vi "简易计算器的制作(下).vi"() -> ()   [LabVIEW 2018]
panel:
  out "结果输出":dbl
  out "当前输入":string
  in  "?":bool
  in  "?":bool
  in  "?":bool
  in  "?":bool
  in  "?":bool
  in  "?":bool
  in  "?":bool
  in  "?":bool
  in  "?":bool
  in  "?":bool
  in  "?":bool
  in  "?":bool
  in  "?":bool
  in  "?":bool
  in  "?":bool
  in  "?":bool
  # "简易计算器"
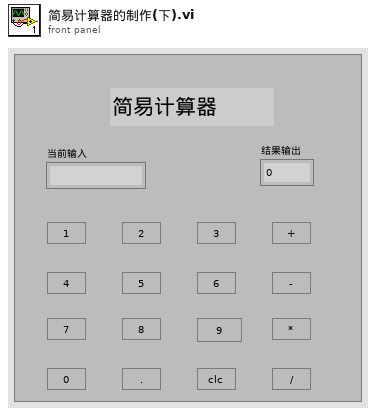
[diagram p1: front panel]
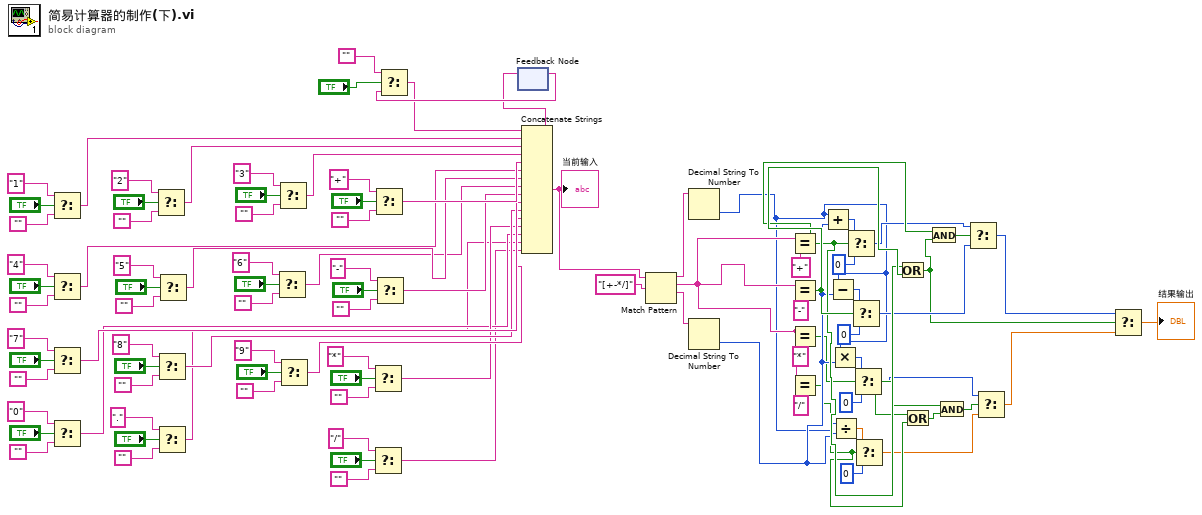
[diagram p0: block diagram]
diagram:
  n1 = Select(t="1", s="?", f="") -> (s? t:f=w53:string)
  n2 = Select(t="4", s="?", f="") -> (s? t:f=w49:string)
  n3 = Select(t="7", s="?", f="") -> (s? t:f=w45:string)
  n4 = Select(t="0", s="?", f="") -> (s? t:f=w41:string)
  n5 = Select(t="2", s="?", f="") -> (s? t:f=w52:string)
  n6 = Select(t="8", s="?", f="") -> (s? t:f=w44:string)
  n7 = Select(t=".", s="?", f="") -> (s? t:f=w40:string)
  n8 = Select(t="5", s="?", f="") -> (s? t:f=w48:string)
  n9 = Select(t="6", s="?", f="") -> (s? t:f=w47:string)
  n10 = Select(t="3", s="?", f="") -> (s? t:f=w51:string)
  n11 = Select(t="9", s="?", f="") -> (s? t:f=w43:string)
  n12 = Select(t="*", s="?", f="") -> (s? t:f=w42:string)
  n13 = Select(t="/", s="?", f="") -> (s? t:f=w39:string)
  n14 = Select(t="+", s="?", f="") -> (s? t:f=w50:string)
  n15 = Select(t="-", s="?", f="") -> (s? t:f=w46:string)
  n16 = feedback #1() -> (w36:string)  [unwired: 1 in]
  n17 = Select(t="", s="?", f=w36) -> (s? t:f=w35:string)
  n18 = Concatenate Strings(w35, w53, w52, w51, w50, w49, w48, w47, w46, w45, w44, w43, w42, w41, w40, w39) -> (w34:string)
  "当前输入" <- w34
  n19 = feedback-in #1(w34) -> ()
  n20 = Match Pattern(string=w34, regular expression="[+-*/]") -> (before substring=w32:string, match substring=w26:string, after substring=w31:string)  [unwired: 1 in, 1 out]
  n21 = Decimal String To Number(string=w32) -> (number=w11:i32)  [unwired: 2 in, 1 out]
  n22 = Decimal String To Number(string=w31) -> (number=w12:i32)  [unwired: 2 in, 1 out]
  n23 = Equal?(x=w26, y="+") -> (x = y?=w16:bool)
  n24 = Equal?(x=w26, y="-") -> (x = y?=w17:bool)
  n25 = Equal?(x=w26, y="*") -> (x = y?=w8:bool)
  n26 = Equal?(x=w26, y="/") -> (x = y?=w10:bool)
  n27 = Add(x=w11, y=w12) -> (x+y=w25:i32)
  n28 = Subtract(x=w11, y=w12) -> (x-y=w23:i32)
  n29 = Multiply(x=w11, y=w12) -> (x*y=w21:i32)
  n30 = Divide(x=w11, y=w12) -> (x/y=w19:dbl)
  n31 = Select(t=w25, s=w16, f=0) -> (s? t:f=w14:i32)
  n32 = Select(t=w23, s=w17, f=0) -> (s? t:f=w13:i32)
  n33 = Select(t=w21, s=w8, f=0) -> (s? t:f=w6:i32)
  n34 = Select(t=w19, s=w10, f=0) -> (s? t:f=w5:dbl)
  n35 = Or(x=w16, y=w17) -> (x .or. y?=w4:bool)
  n36 = Or(x=w8, y=w10) -> (x .or. y?=w9:bool)
  n37 = And(x=w16, y=w4) -> (x .and. y?=w15:bool)
  n38 = And(x=w8, y=w9) -> (x .and. y?=w7:bool)
  n39 = Select(t=w14, s=w15, f=w13) -> (s? t:f=w3:i32)
  n40 = Select(t=w6, s=w7, f=w5) -> (s? t:f=w2:dbl)
  n41 = Select(t=w3, s=w4, f=w2) -> (s? t:f=→"结果输出":dbl)
